vi "getDistFolderPath.vi"() -> (0 "Dist Folder Path":path)   [LabVIEW 2017, in "shared.lvlib"]
uses:
  shared.lvlib
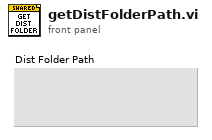
[diagram p1: front panel]
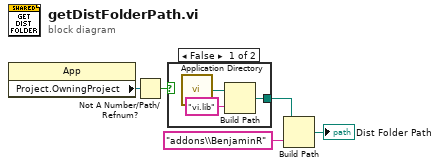
[diagram p0: block diagram]
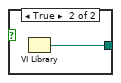
[diagram p2: hidden frame]
diagram:
  n1 = property class="App"() -> ("Project.OwningProject"=w2:refnum<vi>)  [unwired: 2 in, 2 out]
  n2 = Not A Number/Path/Refnum?(number/path/refnum=w2) -> (NaN/Path/Refnum?=w3:bool)
  n3 = case shown="False" w3 {
    tunnel: [w7 w9] -> w1
    frame False {
      n4 = call <vilib>:"Application Directory.vi"() -> ("Application Directory"=w8:path)
      n5 = Build Path(base path=w8, name or relative path="vi.lib") -> (appended path=w7:path)
    }
    frame True {
      n6 = VI Library() -> (path=w9:path)
    }
  }
  n7 = Build Path(base path=w1, name or relative path="addons\\BenjaminR") -> (appended path=→"Dist Folder Path":path)
